vi "Get Current Peak High Limit.vi"(0 "VISA resource name":refnum<visa-resource-name>, 11 "error in (no error)":errorcluster) -> (4 "VISA resource name out":refnum<visa-resource-name>, 6 "Current Peak High Limit (A)":dbl, 15 "error out":errorcluster)   [LabVIEW 2016, in "APT 300XAC Series.lvlib"]
doc: "Gets the Current Peak high limit set to the active step of the Power source instrument."
uses:
  APT 300XAC Series.lvlib
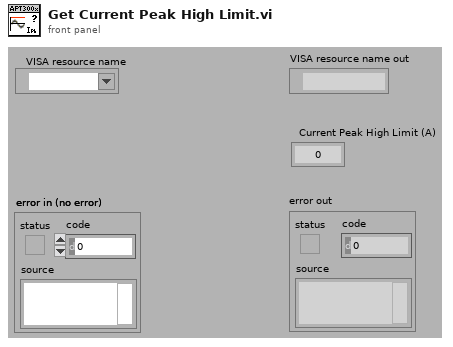
[diagram p1: front panel]
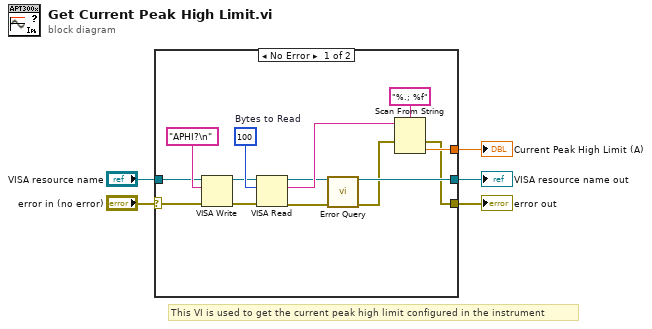
[diagram p0: block diagram]
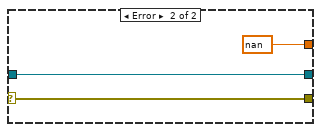
[diagram p2: hidden frame]
diagram:
  # "This VI is used to get the current peak high limit configured in the instrument"
  n1 = case shown="No Error" "error in (no error)" {
    selector: "error in (no error)" -> [w15 w22]
    tunnel: [w6 w22] -> w4
    tunnel: [w10 w21] -> w2
    tunnel: "VISA resource name" -> [w14 w21]
    tunnel: [w11 nan] -> w1
    frame No Error {
      w19 = u32 100  # Bytes to Read
      n2 = VISA Write(VISA resource name=w14, write buffer="APHI?\n", error in (no error)=w15) -> (VISA resource name out=w17:refnum<visa-resource-name>, error out=w18:errorcluster)  [unwired: 1 out]
      n3 = VISA Read(VISA resource name=w17, byte count=w19, error in (no error)=w18) -> (VISA resource name out=w9:refnum<visa-resource-name>, read buffer=w13:string, error out=w8:errorcluster)  [unwired: 1 out]
      n4 = call "Error Query.vi"("VISA resource name"=w9, "error in (no error)"=w8) -> ("VISA resource name out"=w10:refnum<visa-resource-name>, "error out"=w7:errorcluster)  [unwired: 10 in, 2 out]
      n5 = Scan From String(format string="%.; %f", input string=w13, error in=w7) -> (error out=w6:errorcluster, output 1=w11:dbl)  [unwired: 2 in, 2 out]
    }
    frame Error {
    }
  }
  "error out" <- w4
  "VISA resource name out" <- w2
  "Current Peak High Limit (A)" <- w1
